vi "AMC_discover_devices_SubVI.vi"() -> (0 "error out":errorcluster, 1 "No. of found devices":i32, 2 "IPs":string[](array[string]), 3 "Found Devices":T1(array[cluster]))   [LabVIEW 2019]
uses:
  attocube-discovery-dll.dll
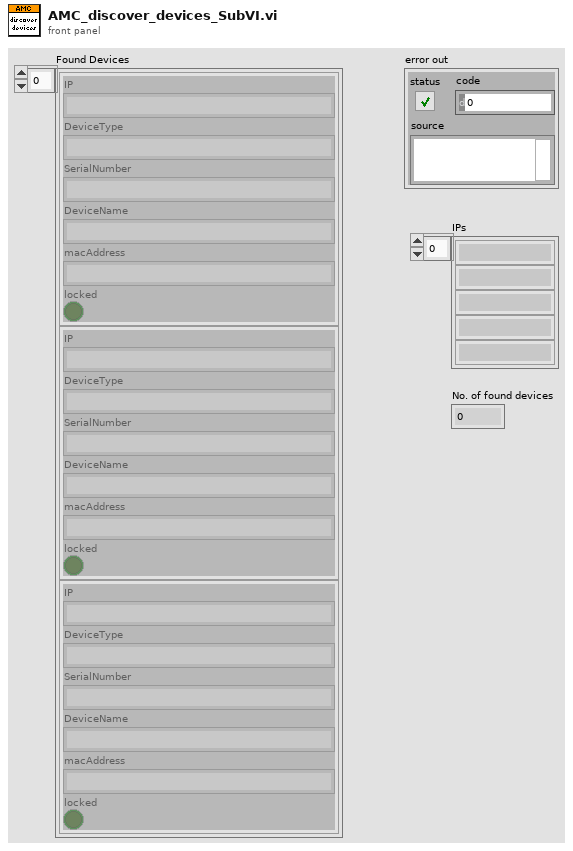
[diagram p1: front panel]
types:
  T1 = cluster{"IP":string, "DeviceType":string, "SerialNumber":string, "DeviceName":string, "macAddress":string, "locked":bool}[]
  T2 = cluster{"macAddress[31]":i8, "macAddress[30]":i8, "macAddress[29]":i8, "macAddress[28]":i8, "macAddress[27]":i8, "macAddress[26]":i8, "macAddress[25]":i8, "macAddress[24]":i8, "macAddress[23]":i8, "macAddress[22]":i8, "macAddress[21]":i8, "macAddress[20]":i8, "macAddress[19]":i8, "macAddress[18]":i8, "macAddress[17]":i8, "macAddress[16]":i8, "macAddress[15]":i8, "macAddress[14]":i8, "macAddress[13]":i8, "macAddress[12]":i8, "macAddress[11]":i8, "macAddress[10]":i8, "macAddress[9]":i8, "macAddress[8]":i8, "macAddress[7]":i8, "macAddress[6]":i8, "macAddress[5]":i8, "macAddress[4]":i8, "macAddress[3]":i8, "macAddress[2]":i8, "macAddress[1]":i8, "macAddress[0]":i8, "deviceName[31]":i8, "deviceName[30]":i8, "deviceName[29]":i8, "deviceName[28]":i8, "deviceName[27]":i8, "deviceName[26]":i8, "deviceName[25]":i8, "deviceName[24]":i8, "deviceName[23]":i8, "deviceName[22]":i8, "deviceName[21]":i8, "deviceName[20]":i8, "deviceName[19]":i8, "deviceName[18]":i8, "deviceName[17]":i8, "deviceName[16]":i8, "deviceName[15]":i8, "deviceName[14]":i8, "deviceName[13]":i8, "deviceName[12]":i8, "deviceName[11]":i8, "deviceName[10]":i8, "deviceName[9]":i8, "deviceName[8]":i8, "deviceName[7]":i8, "deviceName[6]":i8, "deviceName[5]":i8, "deviceName[4]":i8, "deviceName[3]":i8, "deviceName[2]":i8, "deviceName[1]":i8, "deviceName[0]":i8, "serialNumber[31]":i8, "serialNumber[30]":i8, "serialNumber[29]":i8, "serialNumber[28]":i8, "serialNumber[27]":i8, "serialNumber[26]":i8, "serialNumber[25]":i8, "serialNumber[24]":i8, "serialNumber[23]":i8, "serialNumber[22]":i8, "serialNumber[21]":i8, "serialNumber[20]":i8, "serialNumber[19]":i8, "serialNumber[18]":i8, "serialNumber[17]":i8, "serialNumber[16]":i8, "serialNumber[15]":i8, "serialNumber[14]":i8, "serialNumber[13]":i8, "serialNumber[12]":i8, "serialNumber[11]":i8, "serialNumber[10]":i8, "serialNumber[9]":i8, "serialNumber[8]":i8, "serialNumber[7]":i8, "serialNumber[6]":i8, "serialNumber[5]":i8, "serialNumber[4]":i8, "serialNumber[3]":i8, "serialNumber[2]":i8, "serialNumber[1]":i8, "serialNumber[0]":i8, "deviceType[31]":i8, "deviceType[30]":i8, "deviceType[29]":i8, "deviceType[28]":i8, "deviceType[27]":i8, "deviceType[26]":i8, "deviceType[25]":i8, "deviceType[24]":i8, "deviceType[23]":i8, "deviceType[22]":i8, "deviceType[21]":i8, "deviceType[20]":i8, "deviceType[19]":i8, "deviceType[18]":i8, "deviceType[17]":i8, "deviceType[16]":i8, "deviceType[15]":i8, "deviceType[14]":i8, "deviceType[13]":i8, "deviceType[12]":i8, "deviceType[11]":i8, "deviceType[10]":i8, "deviceType[9]":i8, "deviceType[8]":i8, "deviceType[7]":i8, "deviceType[6]":i8, "deviceType[5]":i8, "deviceType[4]":i8, "deviceType[3]":i8, "deviceType[2]":i8, "deviceType[1]":i8, "deviceType[0]":i8, "ipAddress[31]":i8, "ipAddress[30]":i8, "ipAddress[29]":i8, "ipAddress[28]":i8, "ipAddress[27]":i8, "ipAddress[26]":i8, "ipAddress[25]":i8, "ipAddress[24]":i8, "ipAddress[23]":i8, "ipAddress[22]":i8, "ipAddress[21]":i8, "ipAddress[20]":i8, "ipAddress[19]":i8, "ipAddress[18]":i8, "ipAddress[17]":i8, "ipAddress[16]":i8, "ipAddress[15]":i8, "ipAddress[14]":i8, "ipAddress[13]":i8, "ipAddress[12]":i8, "ipAddress[11]":i8, "ipAddress[10]":i8, "ipAddress[9]":i8, "ipAddress[8]":i8, "ipAddress[7]":i8, "ipAddress[6]":i8, "ipAddress[5]":i8, "ipAddress[4]":i8, "ipAddress[3]":i8, "ipAddress[2]":i8, "ipAddress[1]":i8, "ipAddress[0]":i8, "locked":bool}
  T3 = cluster{"macAddress[31]":i8, "macAddress[30]":i8, "macAddress[29]":i8, "macAddress[28]":i8, "macAddress[27]":i8, "macAddress[26]":i8, "macAddress[25]":i8, "macAddress[24]":i8, "macAddress[23]":i8, "macAddress[22]":i8, "macAddress[21]":i8, "macAddress[20]":i8, "macAddress[19]":i8, "macAddress[18]":i8, "macAddress[17]":i8, "macAddress[16]":i8, "macAddress[15]":i8, "macAddress[14]":i8, "macAddress[13]":i8, "macAddress[12]":i8, "macAddress[11]":i8, "macAddress[10]":i8, "macAddress[9]":i8, "macAddress[8]":i8, "macAddress[7]":i8, "macAddress[6]":i8, "macAddress[5]":i8, "macAddress[4]":i8, "macAddress[3]":i8, "macAddress[2]":i8, "macAddress[1]":i8, "macAddress[0]":i8}
  T4 = cluster{"deviceName[31]":i8, "deviceName[30]":i8, "deviceName[29]":i8, "deviceName[28]":i8, "deviceName[27]":i8, "deviceName[26]":i8, "deviceName[25]":i8, "deviceName[24]":i8, "deviceName[23]":i8, "deviceName[22]":i8, "deviceName[21]":i8, "deviceName[20]":i8, "deviceName[19]":i8, "deviceName[18]":i8, "deviceName[17]":i8, "deviceName[16]":i8, "deviceName[15]":i8, "deviceName[14]":i8, "deviceName[13]":i8, "deviceName[12]":i8, "deviceName[11]":i8, "deviceName[10]":i8, "deviceName[9]":i8, "deviceName[8]":i8, "deviceName[7]":i8, "deviceName[6]":i8, "deviceName[5]":i8, "deviceName[4]":i8, "deviceName[3]":i8, "deviceName[2]":i8, "deviceName[1]":i8, "deviceName[0]":i8}
  T5 = cluster{"serialNumber[31]":i8, "serialNumber[30]":i8, "serialNumber[29]":i8, "serialNumber[28]":i8, "serialNumber[27]":i8, "serialNumber[26]":i8, "serialNumber[25]":i8, "serialNumber[24]":i8, "serialNumber[23]":i8, "serialNumber[22]":i8, "serialNumber[21]":i8, "serialNumber[20]":i8, "serialNumber[19]":i8, "serialNumber[18]":i8, "serialNumber[17]":i8, "serialNumber[16]":i8, "serialNumber[15]":i8, "serialNumber[14]":i8, "serialNumber[13]":i8, "serialNumber[12]":i8, "serialNumber[11]":i8, "serialNumber[10]":i8, "serialNumber[9]":i8, "serialNumber[8]":i8, "serialNumber[7]":i8, "serialNumber[6]":i8, "serialNumber[5]":i8, "serialNumber[4]":i8, "serialNumber[3]":i8, "serialNumber[2]":i8, "serialNumber[1]":i8, "serialNumber[0]":i8}
  T6 = cluster{"deviceType[31]":i8, "deviceType[30]":i8, "deviceType[29]":i8, "deviceType[28]":i8, "deviceType[27]":i8, "deviceType[26]":i8, "deviceType[25]":i8, "deviceType[24]":i8, "deviceType[23]":i8, "deviceType[22]":i8, "deviceType[21]":i8, "deviceType[20]":i8, "deviceType[19]":i8, "deviceType[18]":i8, "deviceType[17]":i8, "deviceType[16]":i8, "deviceType[15]":i8, "deviceType[14]":i8, "deviceType[13]":i8, "deviceType[12]":i8, "deviceType[11]":i8, "deviceType[10]":i8, "deviceType[9]":i8, "deviceType[8]":i8, "deviceType[7]":i8, "deviceType[6]":i8, "deviceType[5]":i8, "deviceType[4]":i8, "deviceType[3]":i8, "deviceType[2]":i8, "deviceType[1]":i8, "deviceType[0]":i8}
  T7 = cluster{"ipAddress[31]":i8, "ipAddress[30]":i8, "ipAddress[29]":i8, "ipAddress[28]":i8, "ipAddress[27]":i8, "ipAddress[26]":i8, "ipAddress[25]":i8, "ipAddress[24]":i8, "ipAddress[23]":i8, "ipAddress[22]":i8, "ipAddress[21]":i8, "ipAddress[20]":i8, "ipAddress[19]":i8, "ipAddress[18]":i8, "ipAddress[17]":i8, "ipAddress[16]":i8, "ipAddress[15]":i8, "ipAddress[14]":i8, "ipAddress[13]":i8, "ipAddress[12]":i8, "ipAddress[11]":i8, "ipAddress[10]":i8, "ipAddress[9]":i8, "ipAddress[8]":i8, "ipAddress[7]":i8, "ipAddress[6]":i8, "ipAddress[5]":i8, "ipAddress[4]":i8, "ipAddress[3]":i8, "ipAddress[2]":i8, "ipAddress[1]":i8, "ipAddress[0]":i8}
  T8 = cluster{"string":string, "string":string, "string":string, "string":string, "string":string, "locked":bool}
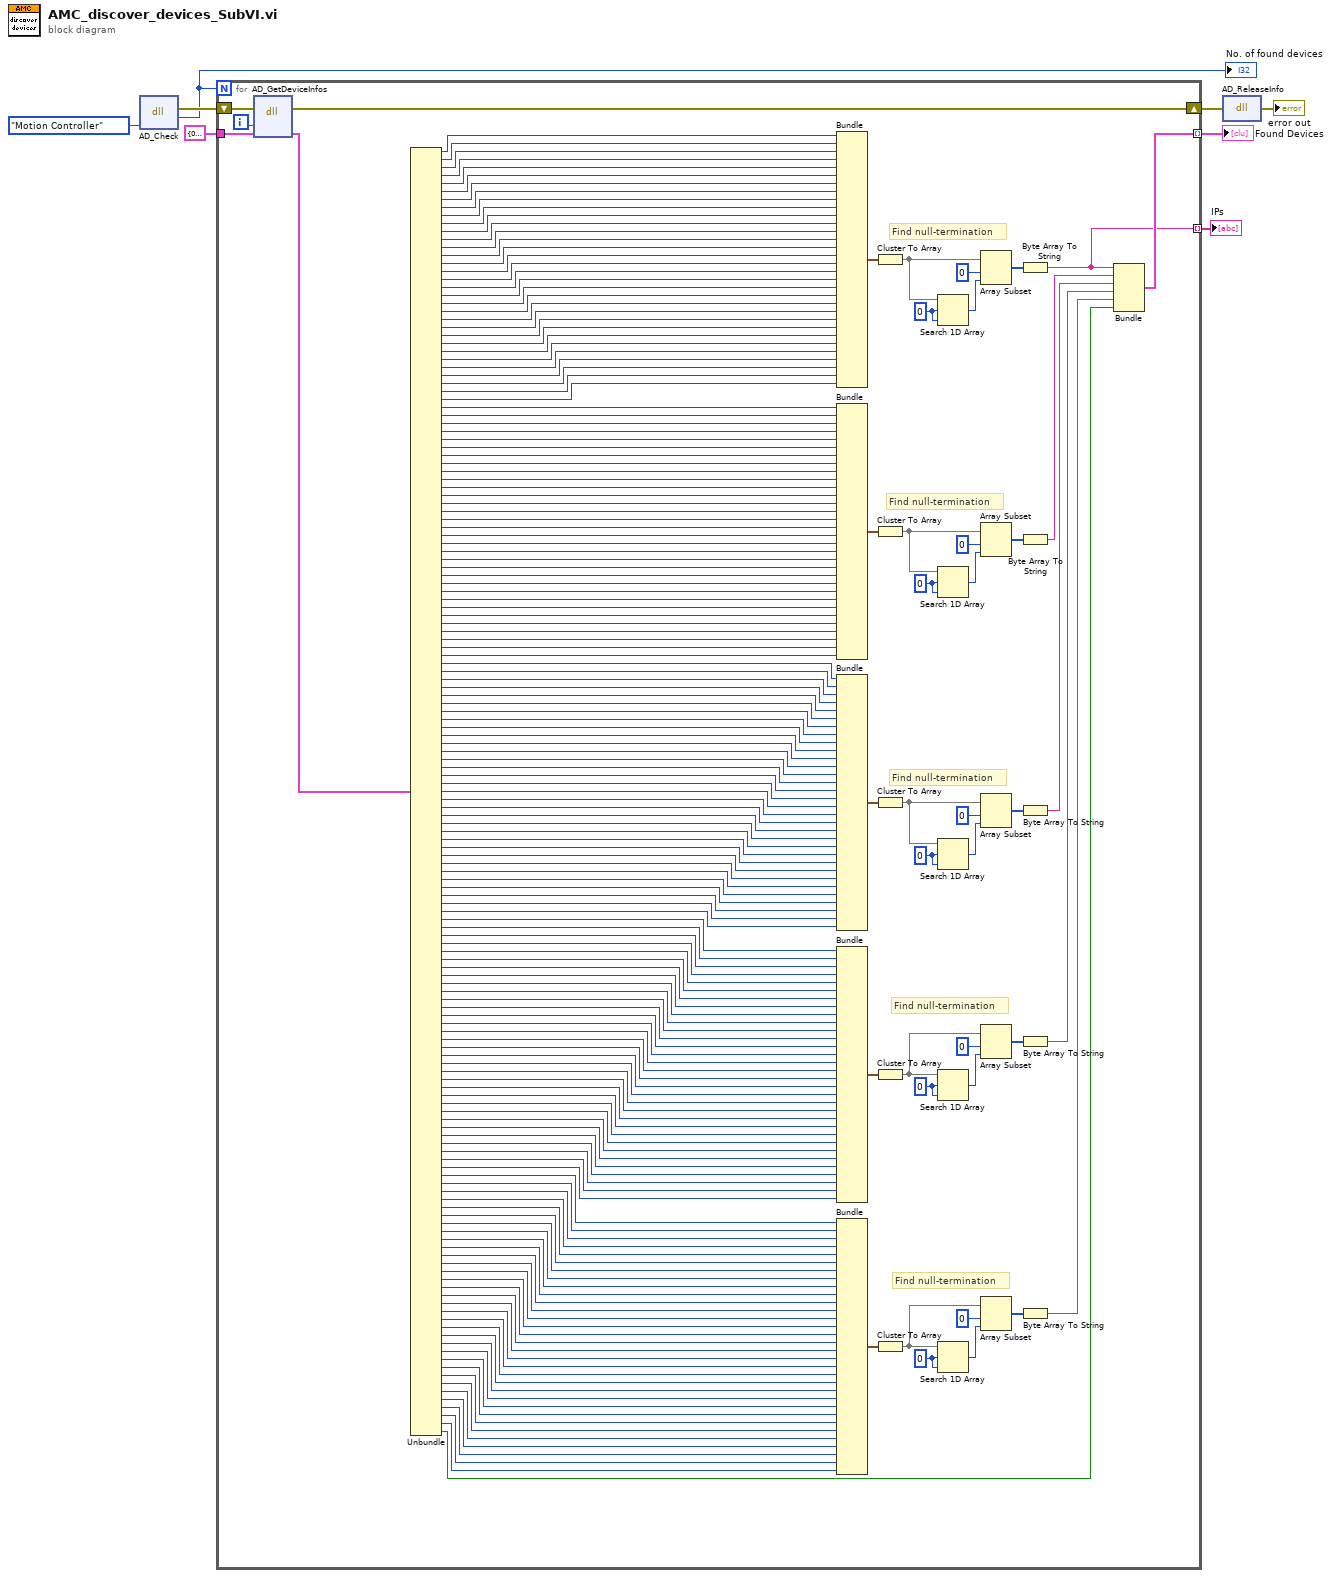
[diagram p0: block diagram]
diagram:
  n1 = dll-call lib="\\\\bob\\Recherche/Morris/Appareils/Attocube/USB Key/AMC100/Software/05_AMC100_LabVIEW_Driver/32bit/Discovery/attocube-discovery-dll.dll" fn="AD_Check"("DeviceType"=enum16{"IDS3010", "Motion Controller", "Both"}."Motion Controller" ("DeviceType to find")) -> (error out=w8:errorcluster, "number_of_found_devices"=w5:i32)  [unwired: 4 in, 1 out]
  "No. of found devices" <- w5
  n2 = for {
    N: w5 -> [_]
    tunnel: T2 {"macAddress[31]"=0, "macAddress[30]"=0, "macAddress[29]"=0, "macAddress[28]"=0, "macAddress[27]"=0, "macAddress[26]"=0, "macAddress[25]"=0, "macAddress[24]"=0, "macAddress[23]"=0, "macAddress[22]"=0, "macAddress[21]"=0, "macAddress[20]"=0, "macAddress[19]"=0, "macAddress[18]"=0, "macAddress[17]"=0, "macAddress[16]"=0, "macAddress[15]"=0, "macAddress[14]"=0, "macAddress[13]"=0, "macAddress[12]"=0, "macAddress[11]"=0, "macAddress[10]"=0, "macAddress[9]"=0, "macAddress[8]"=0, "macAddress[7]"=0, "macAddress[6]"=0, "macAddress[5]"=0, "macAddress[4]"=0, "macAddress[3]"=0, "macAddress[2]"=0, "macAddress[1]"=0, "macAddress[0]"=0, "deviceName[31]"=0, "deviceName[30]"=0, "deviceName[29]"=0, "deviceName[28]"=0, "deviceName[27]"=0, "deviceName[26]"=0, "deviceName[25]"=0, "deviceName[24]"=0, "deviceName[23]"=0, "deviceName[22]"=0, "deviceName[21]"=0, "deviceName[20]"=0, "deviceName[19]"=0, "deviceName[18]"=0, "deviceName[17]"=0, "deviceName[16]"=0, "deviceName[15]"=0, "deviceName[14]"=0, "deviceName[13]"=0, "deviceName[12]"=0, "deviceName[11]"=0, "deviceName[10]"=0, "deviceName[9]"=0, "deviceName[8]"=0, "deviceName[7]"=0, "deviceName[6]"=0, "deviceName[5]"=0, "deviceName[4]"=0, "deviceName[3]"=0, "deviceName[2]"=0, "deviceName[1]"=0, "deviceName[0]"=0, "serialNumber[31]"=0, "serialNumber[30]"=0, "serialNumber[29]"=0, "serialNumber[28]"=0, "serialNumber[27]"=0, "serialNumber[26]"=0, "serialNumber[25]"=0, "serialNumber[24]"=0, "serialNumber[23]"=0, "serialNumber[22]"=0, "serialNumber[21]"=0, "serialNumber[20]"=0, "serialNumber[19]"=0, "serialNumber[18]"=0, "serialNumber[17]"=0, "serialNumber[16]"=0, "serialNumber[15]"=0, "serialNumber[14]"=0, "serialNumber[13]"=0, "serialNumber[12]"=0, "serialNumber[11]"=0, "serialNumber[10]"=0, "serialNumber[9]"=0, "serialNumber[8]"=0, "serialNumber[7]"=0, "serialNumber[6]"=0, "serialNumber[5]"=0, "serialNumber[4]"=0, "serialNumber[3]"=0, "serialNumber[2]"=0, "serialNumber[1]"=0, "serialNumber[0]"=0, "deviceType[31]"=0, "deviceType[30]"=0, "deviceType[29]"=0, "deviceType[28]"=0, "deviceType[27]"=0, "deviceType[26]"=0, "deviceType[25]"=0, "deviceType[24]"=0, "deviceType[23]"=0, "deviceType[22]"=0, "deviceType[21]"=0, "deviceType[20]"=0, "deviceType[19]"=0, "deviceType[18]"=0, "deviceType[17]"=0, "deviceType[16]"=0, "deviceType[15]"=0, "deviceType[14]"=0, "deviceType[13]"=0, "deviceType[12]"=0, "deviceType[11]"=0, "deviceType[10]"=0, "deviceType[9]"=0, "deviceType[8]"=0, "deviceType[7]"=0, "deviceType[6]"=0, "deviceType[5]"=0, "deviceType[4]"=0, "deviceType[3]"=0, "deviceType[2]"=0, "deviceType[1]"=0, "deviceType[0]"=0, "ipAddress[31]"=0, "ipAddress[30]"=0, "ipAddress[29]"=0, "ipAddress[28]"=0, "ipAddress[27]"=0, "ipAddress[26]"=0, "ipAddress[25]"=0, "ipAddress[24]"=0, "ipAddress[23]"=0, "ipAddress[22]"=0, "ipAddress[21]"=0, "ipAddress[20]"=0, "ipAddress[19]"=0, "ipAddress[18]"=0, "ipAddress[17]"=0, "ipAddress[16]"=0, "ipAddress[15]"=0, "ipAddress[14]"=0, "ipAddress[13]"=0, "ipAddress[12]"=0, "ipAddress[11]"=0, "ipAddress[10]"=0, "ipAddress[9]"=0, "ipAddress[8]"=0, "ipAddress[7]"=0, "ipAddress[6]"=0, "ipAddress[5]"=0, "ipAddress[4]"=0, "ipAddress[3]"=0, "ipAddress[2]"=0, "ipAddress[1]"=0, "ipAddress[0]"=0, "locked"=FALSE} ("Original Cluster") -> [w208]
    shift-right: [w209] -> w7
    shift-left: w8 -> [w210]
    tunnel: [w11] -> w4 mode=indexing
    tunnel: [w9] -> w1 mode=indexing
    i -> [w207]
    w19 = i8 0 ("element")
    w26 = i8 0 ("element")
    w33 = i8 0 ("element")
    w39 = i8 0 ("element")
    w43 = i8 0 ("element")
    # "Find null-termination"
    # "Find null-termination"
    # "Find null-termination"
    # "Find null-termination"
    # "Find null-termination"
    n3 = dll-call lib="\\\\bob\\Recherche/Morris/Appareils/Attocube/USB Key/AMC100/Software/05_AMC100_LabVIEW_Driver/32bit/Discovery/attocube-discovery-dll.dll" fn="AD_GetDeviceInfos"(error in=w210, "DeviceIndex"=w207, "DeviceInfo"=w208) -> (error out=w209:errorcluster, "DeviceInfo"=w12:T2)  [unwired: 4 in, 1 out]
    n4 = Unbundle(w12) -> ("macAddress[31]"=w206:i8, "macAddress[30]"=w205:i8, "macAddress[29]"=w204:i8, "macAddress[28]"=w203:i8, "macAddress[27]"=w202:i8, "macAddress[26]"=w201:i8, "macAddress[25]"=w200:i8, "macAddress[24]"=w199:i8, "macAddress[23]"=w198:i8, "macAddress[22]"=w197:i8, "macAddress[21]"=w196:i8, "macAddress[20]"=w194:i8, "macAddress[19]"=w193:i8, "macAddress[18]"=w192:i8, "macAddress[17]"=w191:i8, "macAddress[16]"=w190:i8, "macAddress[15]"=w189:i8, "macAddress[14]"=w188:i8, "macAddress[13]"=w187:i8, "macAddress[12]"=w186:i8, "macAddress[11]"=w185:i8, "macAddress[10]"=w184:i8, "macAddress[9]"=w183:i8, "macAddress[8]"=w182:i8, "macAddress[7]"=w181:i8, "macAddress[6]"=w180:i8, "macAddress[5]"=w179:i8, "macAddress[4]"=w178:i8, "macAddress[3]"=w177:i8, "macAddress[2]"=w176:i8, "macAddress[1]"=w175:i8, "macAddress[0]"=w174:i8, "deviceName[31]"=w173:i8, "deviceName[30]"=w172:i8, "deviceName[29]"=w171:i8, "deviceName[28]"=w170:i8, "deviceName[27]"=w169:i8, "deviceName[26]"=w168:i8, "deviceName[25]"=w167:i8, "deviceName[24]"=w166:i8, "deviceName[23]"=w165:i8, "deviceName[22]"=w164:i8, "deviceName[21]"=w163:i8, "deviceName[20]"=w162:i8, "deviceName[19]"=w161:i8, "deviceName[18]"=w160:i8, "deviceName[17]"=w159:i8, "deviceName[16]"=w158:i8, "deviceName[15]"=w157:i8, "deviceName[14]"=w156:i8, "deviceName[13]"=w155:i8, "deviceName[12]"=w154:i8, "deviceName[11]"=w153:i8, "deviceName[10]"=w152:i8, "deviceName[9]"=w151:i8, "deviceName[8]"=w150:i8, "deviceName[7]"=w149:i8, "deviceName[6]"=w148:i8, "deviceName[5]"=w147:i8, "deviceName[4]"=w146:i8, "deviceName[3]"=w145:i8, "deviceName[2]"=w144:i8, "deviceName[1]"=w143:i8, "deviceName[0]"=w142:i8, "serialNumber[31]"=w141:i8, "serialNumber[30]"=w140:i8, "serialNumber[29]"=w139:i8, "serialNumber[28]"=w138:i8, "serialNumber[27]"=w137:i8, "serialNumber[26]"=w136:i8, "serialNumber[25]"=w135:i8, "serialNumber[24]"=w134:i8, "serialNumber[23]"=w133:i8, "serialNumber[22]"=w132:i8, "serialNumber[21]"=w131:i8, "serialNumber[20]"=w130:i8, "serialNumber[19]"=w129:i8, "serialNumber[18]"=w128:i8, "serialNumber[17]"=w127:i8, "serialNumber[16]"=w126:i8, "serialNumber[15]"=w125:i8, "serialNumber[14]"=w124:i8, "serialNumber[13]"=w123:i8, "serialNumber[12]"=w122:i8, "serialNumber[11]"=w121:i8, "serialNumber[10]"=w120:i8, "serialNumber[9]"=w119:i8, "serialNumber[8]"=w118:i8, "serialNumber[7]"=w117:i8, "serialNumber[6]"=w116:i8, "serialNumber[5]"=w115:i8, "serialNumber[4]"=w114:i8, "serialNumber[3]"=w113:i8, "serialNumber[2]"=w112:i8, "serialNumber[1]"=w111:i8, "serialNumber[0]"=w110:i8, "deviceType[31]"=w109:i8, "deviceType[30]"=w108:i8, "deviceType[29]"=w107:i8, "deviceType[28]"=w106:i8, "deviceType[27]"=w105:i8, "deviceType[26]"=w104:i8, "deviceType[25]"=w103:i8, "deviceType[24]"=w102:i8, "deviceType[23]"=w101:i8, "deviceType[22]"=w100:i8, "deviceType[21]"=w99:i8, "deviceType[20]"=w98:i8, "deviceType[19]"=w97:i8, "deviceType[18]"=w96:i8, "deviceType[17]"=w95:i8, "deviceType[16]"=w94:i8, "deviceType[15]"=w93:i8, "deviceType[14]"=w92:i8, "deviceType[13]"=w91:i8, "deviceType[12]"=w90:i8, "deviceType[11]"=w89:i8, "deviceType[10]"=w88:i8, "deviceType[9]"=w87:i8, "deviceType[8]"=w86:i8, "deviceType[7]"=w85:i8, "deviceType[6]"=w84:i8, "deviceType[5]"=w83:i8, "deviceType[4]"=w82:i8, "deviceType[3]"=w81:i8, "deviceType[2]"=w80:i8, "deviceType[1]"=w79:i8, "deviceType[0]"=w78:i8, "ipAddress[31]"=w77:i8, "ipAddress[30]"=w76:i8, "ipAddress[29]"=w75:i8, "ipAddress[28]"=w74:i8, "ipAddress[27]"=w73:i8, "ipAddress[26]"=w72:i8, "ipAddress[25]"=w71:i8, "ipAddress[24]"=w70:i8, "ipAddress[23]"=w69:i8, "ipAddress[22]"=w68:i8, "ipAddress[21]"=w67:i8, "ipAddress[20]"=w66:i8, "ipAddress[19]"=w65:i8, "ipAddress[18]"=w64:i8, "ipAddress[17]"=w63:i8, "ipAddress[16]"=w62:i8, "ipAddress[15]"=w61:i8, "ipAddress[14]"=w60:i8, "ipAddress[13]"=w59:i8, "ipAddress[12]"=w58:i8, "ipAddress[11]"=w57:i8, "ipAddress[10]"=w56:i8, "ipAddress[9]"=w55:i8, "ipAddress[8]"=w54:i8, "ipAddress[7]"=w53:i8, "ipAddress[6]"=w52:i8, "ipAddress[5]"=w51:i8, "ipAddress[4]"=w50:i8, "ipAddress[3]"=w49:i8, "ipAddress[2]"=w48:i8, "ipAddress[1]"=w47:i8, "ipAddress[0]"=w46:i8, "locked"=w44:bool)
    n5 = Bundle("macAddress[31]"=w206, "macAddress[30]"=w205, "macAddress[29]"=w204, "macAddress[28]"=w203, "macAddress[27]"=w202, "macAddress[26]"=w201, "macAddress[25]"=w200, "macAddress[24]"=w199, "macAddress[23]"=w198, "macAddress[22]"=w197, "macAddress[21]"=w196, "macAddress[20]"=w194, "macAddress[19]"=w193, "macAddress[18]"=w192, "macAddress[17]"=w191, "macAddress[16]"=w190, "macAddress[15]"=w189, "macAddress[14]"=w188, "macAddress[13]"=w187, "macAddress[12]"=w186, "macAddress[11]"=w185, "macAddress[10]"=w184, "macAddress[9]"=w183, "macAddress[8]"=w182, "macAddress[7]"=w181, "macAddress[6]"=w180, "macAddress[5]"=w179, "macAddress[4]"=w178, "macAddress[3]"=w177, "macAddress[2]"=w176, "macAddress[1]"=w175, "macAddress[0]"=w174) -> (w195:T3)  [unwired: 1 in]
    n6 = Bundle("deviceName[31]"=w173, "deviceName[30]"=w172, "deviceName[29]"=w171, "deviceName[28]"=w170, "deviceName[27]"=w169, "deviceName[26]"=w168, "deviceName[25]"=w167, "deviceName[24]"=w166, "deviceName[23]"=w165, "deviceName[22]"=w164, "deviceName[21]"=w163, "deviceName[20]"=w162, "deviceName[19]"=w161, "deviceName[18]"=w160, "deviceName[17]"=w159, "deviceName[16]"=w158, "deviceName[15]"=w157, "deviceName[14]"=w156, "deviceName[13]"=w155, "deviceName[12]"=w154, "deviceName[11]"=w153, "deviceName[10]"=w152, "deviceName[9]"=w151, "deviceName[8]"=w150, "deviceName[7]"=w149, "deviceName[6]"=w148, "deviceName[5]"=w147, "deviceName[4]"=w146, "deviceName[3]"=w145, "deviceName[2]"=w144, "deviceName[1]"=w143, "deviceName[0]"=w142) -> (w45:T4)  [unwired: 1 in]
    n7 = Bundle("serialNumber[31]"=w141, "serialNumber[30]"=w140, "serialNumber[29]"=w139, "serialNumber[28]"=w138, "serialNumber[27]"=w137, "serialNumber[26]"=w136, "serialNumber[25]"=w135, "serialNumber[24]"=w134, "serialNumber[23]"=w133, "serialNumber[22]"=w132, "serialNumber[21]"=w131, "serialNumber[20]"=w130, "serialNumber[19]"=w129, "serialNumber[18]"=w128, "serialNumber[17]"=w127, "serialNumber[16]"=w126, "serialNumber[15]"=w125, "serialNumber[14]"=w124, "serialNumber[13]"=w123, "serialNumber[12]"=w122, "serialNumber[11]"=w121, "serialNumber[10]"=w120, "serialNumber[9]"=w119, "serialNumber[8]"=w118, "serialNumber[7]"=w117, "serialNumber[6]"=w116, "serialNumber[5]"=w115, "serialNumber[4]"=w114, "serialNumber[3]"=w113, "serialNumber[2]"=w112, "serialNumber[1]"=w111, "serialNumber[0]"=w110) -> (w28:T5)  [unwired: 1 in]
    n8 = Bundle("deviceType[31]"=w109, "deviceType[30]"=w108, "deviceType[29]"=w107, "deviceType[28]"=w106, "deviceType[27]"=w105, "deviceType[26]"=w104, "deviceType[25]"=w103, "deviceType[24]"=w102, "deviceType[23]"=w101, "deviceType[22]"=w100, "deviceType[21]"=w99, "deviceType[20]"=w98, "deviceType[19]"=w97, "deviceType[18]"=w96, "deviceType[17]"=w95, "deviceType[16]"=w94, "deviceType[15]"=w93, "deviceType[14]"=w92, "deviceType[13]"=w91, "deviceType[12]"=w90, "deviceType[11]"=w89, "deviceType[10]"=w88, "deviceType[9]"=w87, "deviceType[8]"=w86, "deviceType[7]"=w85, "deviceType[6]"=w84, "deviceType[5]"=w83, "deviceType[4]"=w82, "deviceType[3]"=w81, "deviceType[2]"=w80, "deviceType[1]"=w79, "deviceType[0]"=w78) -> (w21:T6)  [unwired: 1 in]
    n9 = Bundle("ipAddress[31]"=w77, "ipAddress[30]"=w76, "ipAddress[29]"=w75, "ipAddress[28]"=w74, "ipAddress[27]"=w73, "ipAddress[26]"=w72, "ipAddress[25]"=w71, "ipAddress[24]"=w70, "ipAddress[23]"=w69, "ipAddress[22]"=w68, "ipAddress[21]"=w67, "ipAddress[20]"=w66, "ipAddress[19]"=w65, "ipAddress[18]"=w64, "ipAddress[17]"=w63, "ipAddress[16]"=w62, "ipAddress[15]"=w61, "ipAddress[14]"=w60, "ipAddress[13]"=w59, "ipAddress[12]"=w58, "ipAddress[11]"=w57, "ipAddress[10]"=w56, "ipAddress[9]"=w55, "ipAddress[8]"=w54, "ipAddress[7]"=w53, "ipAddress[6]"=w52, "ipAddress[5]"=w51, "ipAddress[4]"=w50, "ipAddress[3]"=w49, "ipAddress[2]"=w48, "ipAddress[1]"=w47, "ipAddress[0]"=w46) -> (w14:T7)  [unwired: 1 in]
    n10 = Cluster To Array(cluster=w195) -> (array=w42:i8[])
    n11 = Cluster To Array(cluster=w45) -> (array=w35:i8[])
    n12 = Cluster To Array(cluster=w28) -> (array=w27:i8[])
    n13 = Cluster To Array(cluster=w21) -> (array=w22:i8[])
    n14 = Cluster To Array(cluster=w14) -> (array=w15:i8[])
    n15 = Search 1D Array(1D array=w42, element=w43, start index (0)=w43) -> (index of element=w40:i32)
    n16 = Search 1D Array(1D array=w35, element=w39, start index (0)=w39) -> (index of element=w37:i32)
    n17 = Search 1D Array(1D array=w27, element=w33, start index (0)=w33) -> (index of element=w31:i32)
    n18 = Search 1D Array(1D array=w22, element=w26, start index (0)=w26) -> (index of element=w24:i32)
    n19 = Search 1D Array(1D array=w15, element=w19, start index (0)=w19) -> (index of element=w17:i32)
    n20 = Array Subset(array=w42, index=0, length=w40) -> (w10:i8[])
    n21 = Array Subset(array=w35, index=0, length=w37) -> (w36:i8[])
    n22 = Array Subset(array=w27, index=0, length=w31) -> (w30:i8[])
    n23 = Array Subset(array=w22, index=0, length=w24) -> (w23:i8[])
    n24 = Array Subset(array=w15, index=0, length=w17) -> (w16:i8[])
    n25 = Byte Array To String(unsigned byte array=w10) -> (string=w9:string)
    n26 = Byte Array To String(unsigned byte array=w36) -> (string=w34:string)
    n27 = Byte Array To String(unsigned byte array=w30) -> (string=w29:string)
    n28 = Byte Array To String(unsigned byte array=w23) -> (string=w20:string)
    n29 = Byte Array To String(unsigned byte array=w16) -> (string=w13:string)
    n30 = Bundle("string"=w9, "string"=w34, "string"=w29, "string"=w20, "string"=w13, "locked"=w44) -> (w11:T8)  [unwired: 1 in]
  }
  "Found Devices" <- w4
  "IPs" <- w1
  n31 = dll-call lib="\\\\bob\\Recherche/Morris/Appareils/Attocube/USB Key/AMC100/Software/05_AMC100_LabVIEW_Driver/32bit/Discovery/attocube-discovery-dll.dll" fn="AD_ReleaseInfo"(error in=w7) -> (error out=→"error out":errorcluster)  [unwired: 3 in, 1 out]
